vi "Determine E-Series Level.vi"(3 "Number of Bands":u8=4 min=3 max=6 step=1, 5 "Tolerance (%)":dbl) -> (1 "E-Series Level":T1)   [LabVIEW 2018]
doc: "Determines the <b>E-Series Level</b> of a resistor based on its <b>Number of Bands</b> and <b>Tolerance (%)</b>.\n\nThe E-Series Level is an internal classification used by the application to determine which E-Series data must be evaluated for the resistor.\n\nThe classification is defined as follows:\n\nE-SERIES LEVEL CLASSIFICATION\n\nBasic : E3, E6 | ±20 % | 3 bands\nLower : E12, E24 | ±10 %, ±5 %, ±2 % | 4 bands\nMiddle : E48 | ±2 % | 5 bands\nHigher : E96 | ±1 % | 5 or 6 bands\nHighest : E192 | ±0.5 %, ±0.25 %, ±0.1 % | 5 or 6 bands\n\nThe resulting <b>E-Series Level</b> identifies the group of E-Series values applicable to the resistor.\n\nThe VI returns the corresponding E-Series Level and provides individual Boolean indicators for Basic, Lower, Middle, Higher, and Highest."
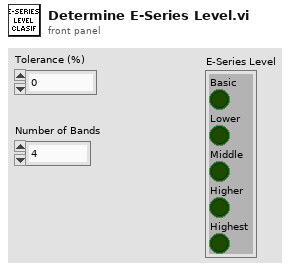
[diagram p1: front panel]
types:
  T1 = cluster{"Basic":bool, "Lower":bool, "Middle":bool, "Higher":bool, "Highest":bool}
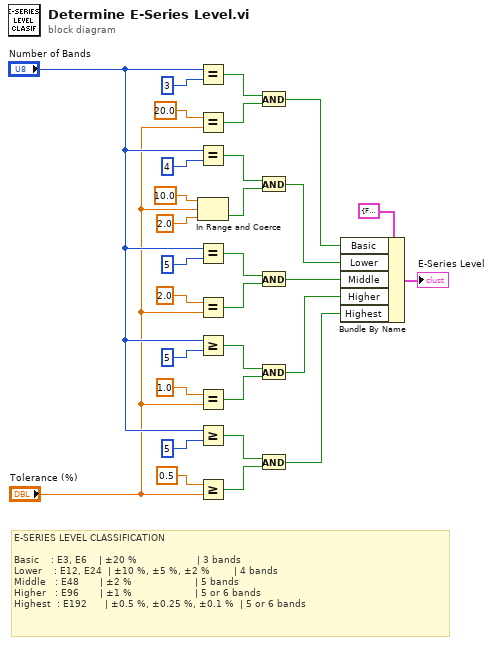
[diagram p0: block diagram]
diagram:
  # "E-SERIES LEVEL CLASSIFICATION\n\nBasic    : E3, E6    | ±20 %                    | 3 bands\nLower    : E12, E24  | ±10 %, ±5 %, ±2 %        | 4 bands\nMiddle   : E48       | ±2 %                     | 5 bands\nHigher   : E96       | ±1 %                     | 5 or 6 bands\nHighest  : E192      | ±0.5 %, ±0.25 %, ±0.1 %  | 5 or 6 bands"
  n1 = Equal?(x="Number of Bands", y=u8 3) -> (x = y?=w2:bool)
  n2 = Equal?(x=20.0, y="Tolerance (%)") -> (x = y?=w3:bool)
  n3 = Equal?(x="Number of Bands", y=u8 4) -> (x = y?=w25:bool)
  n4 = In Range and Coerce(upper limit=10.0 ("x"), x="Tolerance (%)", lower limit=2.0) -> (In Range?=w26:bool)  [unwired: 1 out]
  n5 = Equal?(x="Number of Bands", y=u8 5) -> (x = y?=w22:bool)
  n6 = Equal?(x=2.0, y="Tolerance (%)") -> (x = y?=w21:bool)
  n7 = Greater Or Equal?(x="Number of Bands", y=u8 5) -> (x >= y?=w18:bool)
  n8 = Equal?(x=1.0, y="Tolerance (%)") -> (x = y?=w17:bool)
  n9 = Greater Or Equal?(x="Number of Bands", y=u8 5) -> (x >= y?=w13:bool)
  n10 = Greater Or Equal?(x=0.5, y="Tolerance (%)") -> (x >= y?=w12:bool)
  n11 = And(x=w2, y=w3) -> (x .and. y?=w1:bool)
  n12 = And(x=w25, y=w26) -> (x .and. y?=w10:bool)
  n13 = And(x=w22, y=w21) -> (x .and. y?=w9:bool)
  n14 = And(x=w18, y=w17) -> (x .and. y?=w8:bool)
  n15 = And(x=w13, y=w12) -> (x .and. y?=w7:bool)
  n16 = Bundle By Name(cluster=T1 {"Basic"=FALSE, "Lower"=FALSE, "Middle"=FALSE, "Higher"=FALSE, "Highest"=FALSE}, "Basic"=w1, "Lower"=w10, "Middle"=w9, "Higher"=w8, "Highest"=w7) -> (→"E-Series Level":T1)
